vi "Read Lux (2).vi"(6 "Error In":errorcluster) -> (0 "Error Out":errorcluster, 3 "lux":dbl)   [LabVIEW 2016]
doc: "This VI is used in the LabVIEW Core 1 & 2 courses.\n\nThis VI simulates taking voltage readings from a DAQ board. Use this VI to replace the DAQ Assistant Express VI in any temperature reading exercises in this course. This VI is used as a subVI in all (Demo) exercises."
uses:
  <vilib>/gmath/NI_Gmath.lvlib
  <vilib>/gmath/statdist.llb/Normal Random.vi
panel:
  # "This VI is a demo version of a VI that reads the voltage on Device 1, channel 0.  When scaled by 100, value can represent temperature."
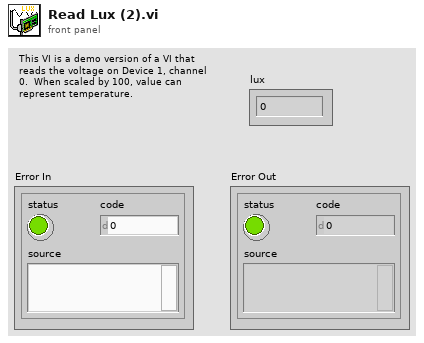
[diagram p1: front panel]
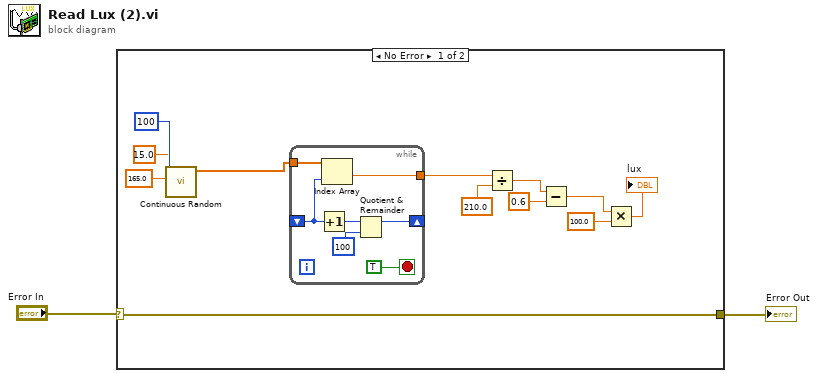
[diagram p0: block diagram]
diagram:
  n1 = case shown="No Error" "Error In" {
    selector: "Error In" -> [w12 w22]
    tunnel: [w12 w22] -> w2
    frame No Error {
      n2 = call-poly <vilib>:"Continuous Random.vi"("std"=15.0, "mean"=165.0, "samples"=100) -> ("normal random data"=w11:dbl[])  [unwired: 7 in, 1 out]
      n3 = while {
        tunnel: w11 -> [w16]
        tunnel: [w17] -> w13
        shift-left: _ -> [w21]
        shift-right: [w18] -> _
        stop <- TRUE stop-if-true
        n4 = Increment(x=w21) -> (x+1=w20:i32)
        n5 = Index Array(array=w16, index=w21) -> (element=w17:dbl)
        n6 = Quotient & Remainder(x=w20, y=100) -> (x-y*floor(x/y)=w18:i32)  [unwired: 1 out]
      }
      n7 = Divide(x=w13, y=210.0) -> (x/y=w4:dbl)
      n8 = Subtract(x=w4, y=0.6) -> (x-y=w5:dbl)
      n9 = Multiply(x=w5, y=100.0) -> (x*y=→"lux":dbl)
    }
    frame Error {
    }
  }
  "Error Out" <- w2
